vi "Combine Two FFTs computed using DIT.vi"(0 "Real FFT 1":fxp<+/-,22,1>, 5 "Imag FFT 1":fxp<+/-,22,1>, 7 "Real FFT 2":fxp<+/-,22,1>, 9 "Imag FFT 2":fxp<+/-,22,1>, 11 "Input Data Valid":bool) -> (4 "Real FFT k":fxp<+/-,24,3> format="%.22g", 6 "Imag FFT k":fxp<+/-,24,3> format="%.22g", 8 "Real FFT k+N/2":fxp<+/-,24,3> format="%.22g", 10 "Imag FFT k+N/2":fxp<+/-,24,3> format="%.22g", 15 "Output Valid":bool)   [LabVIEW 2011]
doc: "This VI combines outputs from two Decimated in Time FFT's and combines them to produce output of original FFT. \n\nReal FFT k, Imag FFT k are the outputs of first half of the spectrum.\nReal FFT k+N/2, Imag FFT k+N/2 are the outputs of fsecond half of the spectrum.\n\n<b> Note: For singled sided- FFT, ignore the second half of the spectrum (leave the outputs unconnected). </b>\n\n<b> Latency = 15 Ticks </b>\n<b> Scaling = 2 </b>\n<b> Resources Used: 1 BRAM, 4 DSP48E Blocks </b>"
uses:
  <vilib>/rvi/FXPMathLib/basic elements/FxpDiscreteDelay/XNode/nifxpmath_DiscreteDelay.xnode
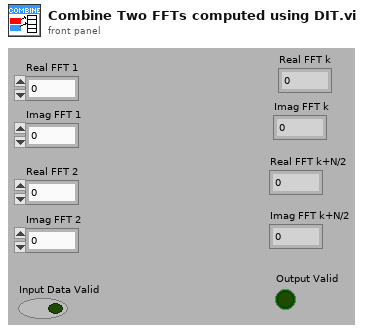
[diagram p1: front panel]
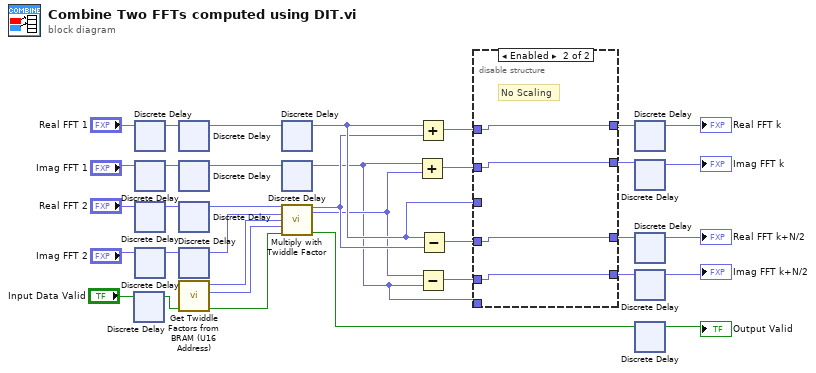
[diagram p0: block diagram]
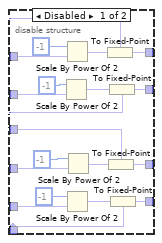
[diagram p2: hidden frame]
diagram:
  n1 = xnode "Discrete Delay"("D"="Input Data Valid") -> ("Q"=w21:bool)
  n2 = xnode "Discrete Delay"("D"="Real FFT 1") -> ("Q"=w17:fxp<+/-,22,1>)
  n3 = xnode "Discrete Delay"("D"="Imag FFT 1") -> ("Q"=w18:fxp<+/-,22,1>)
  n4 = xnode "Discrete Delay"("D"="Real FFT 2") -> ("Q"=w19:fxp<+/-,22,1>)
  n5 = xnode "Discrete Delay"("D"="Imag FFT 2") -> ("Q"=w20:fxp<+/-,22,1>)
  n6 = xnode "Discrete Delay"("D"=w17) -> ("Q"=w31:fxp<+/-,22,1>)
  n7 = xnode "Discrete Delay"("D"=w18) -> ("Q"=w32:fxp<+/-,22,1>)
  n8 = xnode "Discrete Delay"("D"=w19) -> ("Q"=w35:fxp<+/-,22,1>)
  n9 = xnode "Discrete Delay"("D"=w20) -> ("Q"=w34:fxp<+/-,22,1>)
  n10 = call <userlib>:"Get Twiddle Factors from BRAM (U16 Address).vi"("Input Data Valid"=w21) -> ("Output Valid"=w33:bool, "sine"=w1:fxp<+/-,18,2>, "cosine"=w2:fxp<+/-,18,2>)  [unwired: 7 in, 1 out]
  n11 = xnode "Discrete Delay"("D"=w31) -> ("Q"=w25:fxp<+/-,22,1>)
  n12 = xnode "Discrete Delay"("D"=w32) -> ("Q"=w8:fxp<+/-,22,1>)
  n13 = call <userlib>:"Multiply with Twiddle Factor.vi"("Real{Input}"=w35, "Imag{Input}"=w34, "Real{Twiddle}"=w2, "Imag{Twiddle}"=w1, "Input Valid"=w33) -> ("Real{Output}"=w24:fxp<+/-,19,2>, "Imag{Output}"=w23:fxp<+/-,19,2>, "Output Valid"=w26:bool)  [unwired: 8 in]
  n14 = Add(x=w8, y=w23) -> (x+y=w10:fxp<+/-,24,3>)
  n15 = Add(x=w25, y=w24) -> (x+y=w11:fxp<+/-,24,3>)
  n16 = Subtract(x=w23, y=w8) -> (x-y=w7:fxp<+/-,24,3>)
  n17 = Subtract(x=w25, y=w24) -> (x-y=w9:fxp<+/-,24,3>)
  n18 = disable-structure shown="Enabled" {
    disable-tunnel: w25 -> [w45 _]
    disable-tunnel: w11 -> [w44 w57]
    disable-tunnel: w10 -> [w43 w56]
    disable-tunnel: w9 -> [w42 w55]
    disable-tunnel: w8 -> [w41 _]
    disable-tunnel: w7 -> [w40 w54]
    disable-tunnel: [w39 w54] -> w6
    disable-tunnel: [w38 w55] -> w5
    disable-tunnel: [w37 w56] -> w4
    disable-tunnel: [w36 w57] -> w3
    frame Disabled {
      n19 = Scale By Power Of 2(n=-1, x=w43) -> (x*2^n=w50:fxp<+/-,24,3>)
      n20 = Scale By Power Of 2(n=-1, x=w44) -> (x*2^n=w51:fxp<+/-,24,3>)
      n21 = Scale By Power Of 2(n=-1, x=w40) -> (x*2^n=w49:fxp<+/-,24,3>)
      n22 = Scale By Power Of 2(n=-1, x=w42) -> (x*2^n=w48:fxp<+/-,24,3>)
      n23 = To Fixed-Point(fixed-point type=w45, number=w51) -> (fixed-point=w36:fxp<+/-,22,1>)
      n24 = To Fixed-Point(fixed-point type=w45, number=w48) -> (fixed-point=w38:fxp<+/-,22,1>)
      n25 = To Fixed-Point(fixed-point type=w41, number=w50) -> (fixed-point=w37:fxp<+/-,22,1>)
      n26 = To Fixed-Point(fixed-point type=w41, number=w49) -> (fixed-point=w39:fxp<+/-,22,1>)
    }
    frame Enabled {
      # "No Scaling"
    }
  }
  n27 = xnode "Discrete Delay"("D"=w3) -> ("Q"=→"Real FFT k":fxp<+/-,24,3>)
  n28 = xnode "Discrete Delay"("D"=w4) -> ("Q"=→"Imag FFT k":fxp<+/-,24,3>)
  n29 = xnode "Discrete Delay"("D"=w5) -> ("Q"=→"Real FFT k+N/2":fxp<+/-,24,3>)
  n30 = xnode "Discrete Delay"("D"=w6) -> ("Q"=→"Imag FFT k+N/2":fxp<+/-,24,3>)
  n31 = xnode "Discrete Delay"("D"=w26) -> ("Q"=→"Output Valid":bool)
